vi "saveImages.vi"(7 "totalImageNumber":i32, 8 "error in (no error)":errorcluster, 9 "U16bit image data":u16[][](array[numeric]), 10 "Path":path, 11 "ProEM_WinX32 in":refnum<class "ProEM_WinX32.lvclass">) -> (0 "error out":errorcluster, 3 "ProEM_WinX32 out":refnum<class "ProEM_WinX32.lvclass">)   [LabVIEW 2011, in "Hardware.lvlib" / "Channels.lvlib" / "ProEM_WinX32.lvclass"]
uses:
  ProEM_WinX32.lvclass
  Camera/Camera.lvclass
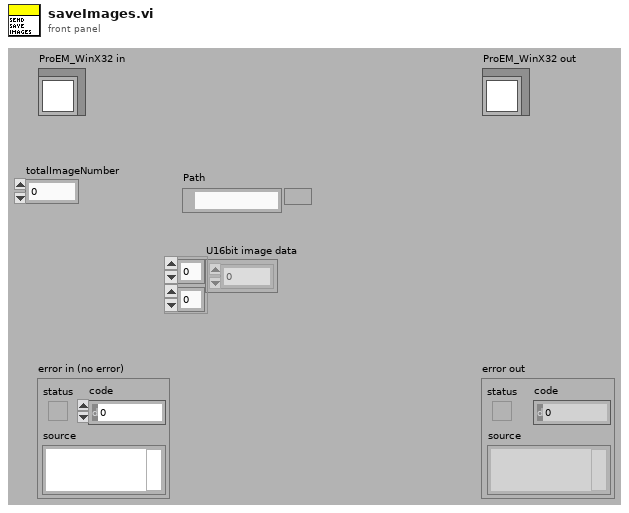
[diagram p1: front panel]
types:
  T1 = cluster{"cameraType":string, "imageName":string, "saved":string, "analysisType":string, "U16bit image data":u16[][], "path":path}
  T2 = typedef "Image Type" = u32
  T3 = typedef "IMAQ Image.ctl" = refnum<image>
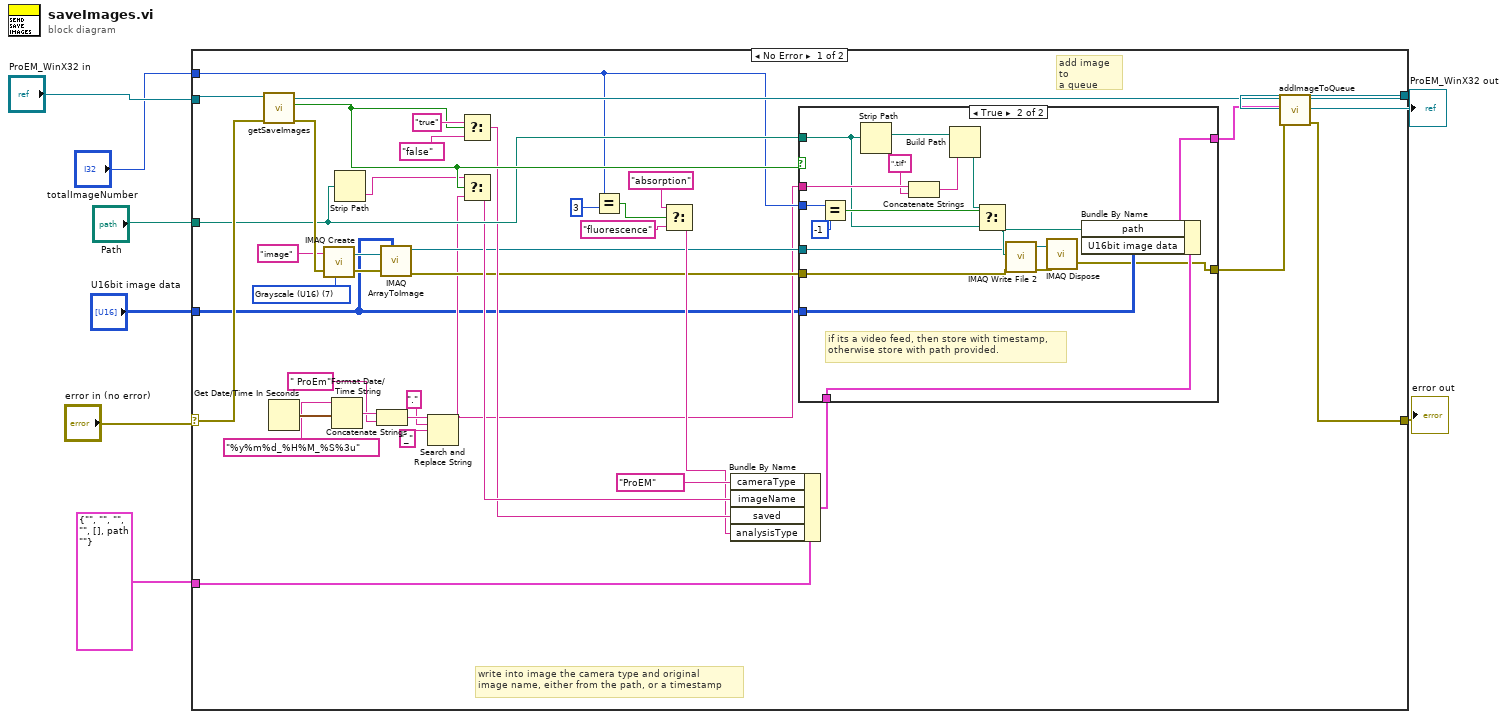
[diagram p0: block diagram]
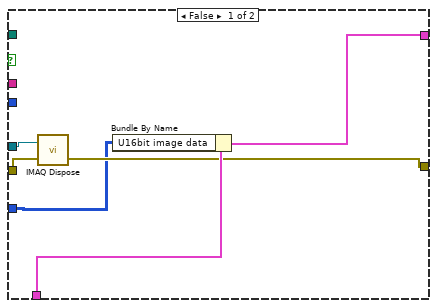
[diagram p2: hidden frame]
diagram:
  n1 = case shown="No Error" "error in (no error)" {
    selector: "error in (no error)" -> [w47 w73]
    tunnel: [w39 w73] -> w6
    tunnel: [w40 w72] -> w5
    tunnel: "ProEM_WinX32 in" -> [w31 w72]
    tunnel: "Path" -> [w25 _]
    tunnel: "U16bit image data" -> [w9 _]
    tunnel: "totalImageNumber" -> [w23 _]
    tunnel: T1 {"cameraType"="", "imageName"="", "saved"="", "analysisType"="", "U16bit image data"=[], "path"=path ""} ("ImageData") -> [w22 _]
    frame No Error {
      w44 = T2 7 items=["Grayscale (U8)", "Grayscale (I16)", "Grayscale (SGL)", "Complex (CSG)", "RGB (U32)", "HSL (U32)", "RGB (U64)", "Grayscale (U16)"] ("Image Type")
      # "write into image the camera type and original\nimage name, either from the path, or a timestamp"
      # "add image to\na queue"
      n2 = call "getSaveImages.vi"("error in (no error)"=w47, "Camera in"=w31) -> ("error out"=w46:errorcluster, "saveImages?"=w26:bool, "Camera out"=w41:refnum<class "ProEM_WinX32.lvclass">)  [unwired: 7 in]
      n3 = Get Date/Time In Seconds() -> (seconds since 1Jan1904=w38:timestamp)
      n4 = call "IMAQ Create"("Image Name"="image", "Image Type"=w44, "error in (no error)"=w46) -> ("New Image"=w43:T3, "error out"=w42:errorcluster)  [unwired: 2 in]
      n5 = Format Date/Time String(time format string (%c)="%y%m%d_%H%M_%S%3u", seconds (now)=w38) -> (date/time string=w36:string)  [unwired: 1 in]
      n6 = Strip Path(path=w25) -> (name=w24:string)  [unwired: 1 out]
      n7 = Concatenate Strings(w36, " ProEm") -> (w13:string)
      n8 = call "IMAQ ArrayToImage"("Image Pixels (U16)"=w9, "error in (no error)"=w42, "Image"=w43) -> ("error out"=w14:errorcluster, "Image Out"=w15:T3)  [unwired: 7 in]
      n9 = Search and Replace String(input string=w13, search string=".", replace string="_") -> (result string=w12:string)  [unwired: 5 in, 3 out]
      n10 = Select(t="true", s=w26, f="false") -> (s? t:f=w19:string)
      n11 = Select(t=w24, s=w26, f=w12) -> (s? t:f=w20:string)
      n12 = Equal?(x=w23, y=3) -> (x = y?=w29:bool)
      n13 = Select(t="absorption", s=w29, f="fluorescence") -> (s? t:f=w18:string)
      n14 = Bundle By Name(cluster=w22, "cameraType"="ProEM", "imageName"=w20, "saved"=w19, "analysisType"=w18) -> (w17:T1)
      n15 = case shown="True" w26 {
        tunnel: [w51 w56] -> w32
        tunnel: [w52 w61] -> w16
        tunnel: w25 -> [_ w64]
        tunnel: w12 -> [_ w70]
        tunnel: w23 -> [_ w63]
        tunnel: w17 -> [w53 w62]
        tunnel: w9 -> [w50 w59]
        tunnel: w15 -> [w49 w55]
        tunnel: w14 -> [w48 w54]
        frame False {
          n16 = call "IMAQ Dispose"("Image"=w49, "error in (no error)"=w48) -> ("error out"=w51:errorcluster)  [unwired: 4 in]
          n17 = Bundle By Name(cluster=w53, "U16bit image data"=w50) -> (w52:T1)
        }
        frame True {
          # "if its a video feed, then store with timestamp,\notherwise store with path provided."
          n18 = Equal?(x=w63, y=-1) -> (x = y?=w65:bool)
          n19 = Strip Path(path=w64) -> (stripped path=w71:path)  [unwired: 1 out]
          n20 = Concatenate Strings(w70, ".tif") -> (w68:string)
          n21 = Build Path(base path=w71, name or relative path=w68) -> (appended path=w66:path)
          n22 = Select(t=w66, s=w65, f=w64) -> (s? t:f=w60:path)
          n23 = call-poly "IMAQ Write File 2"("error in (no error)"=w54, "File Path"=w60, "Image"=w55) -> ("error out"=w58:errorcluster, "Image Out (duplicate)"=w57:T3)  [unwired: 7 in]
          n24 = call "IMAQ Dispose"("Image"=w57, "error in (no error)"=w58) -> ("error out"=w56:errorcluster)  [unwired: 4 in]
          n25 = Bundle By Name(cluster=w62, "path"=w60, "U16bit image data"=w59) -> (w61:T1)
        }
      }
      n26 = call "addImageToQueue.vi"("error in (no error)"=w32, "ImageData"=w16, "Camera in"=w41) -> ("error out"=w39:errorcluster, "Camera out"=w40:refnum<class "ProEM_WinX32.lvclass">)  [unwired: 7 in]
    }
    frame Error {
    }
  }
  "error out" <- w6
  "ProEM_WinX32 out" <- w5
